vi "Batchify All Data.vi"(10 "Data":dbl[][](array[numeric])) -> (2 "Data Out":dbl[][](array[numeric]))   [LabVIEW 2013]
uses:
  Global Data/Names/Source Group Type.ctl
  Offsets Widget/Cartesian Or Actuator.ctl
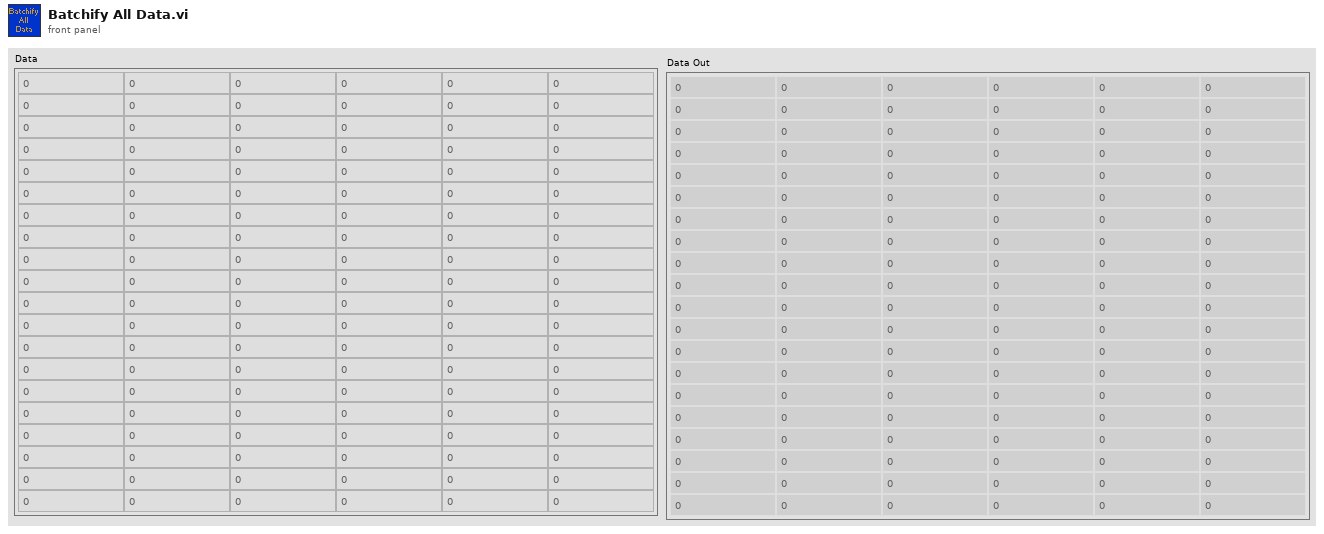
[diagram p1: front panel]
types:
  T1 = typedef "Source Group Type.ctl" = enum16{"LBCB1", "LBCB2", "Consolidated", "External"}
  T2 = typedef "Cartesian Or Actuator.ctl" = bool
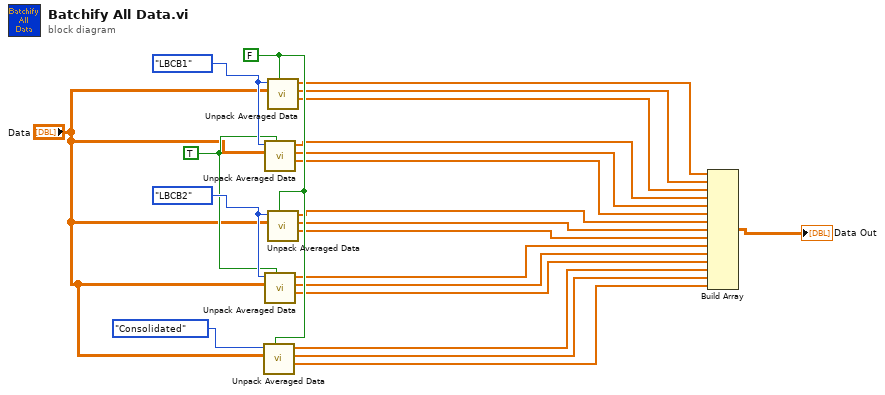
[diagram p0: block diagram]
diagram:
  w21 = Source_Group_Type."LBCB2" ("Source Group")
  w20 = T2 TRUE ("Coordinate Space")
  w18 = T2 FALSE ("Coordinate Space")
  w22 = Source_Group_Type."LBCB1" ("Source Group")
  n1 = call "Unpack Averaged Data.vi"("Coordinate Space"=w18, "Data"="Data", "Source Group"=Source_Group_Type."Consolidated") -> ("Forces"=w2:dbl[], "Disp"=w3:dbl[], "Cmds"=w4:dbl[])  [unwired: 6 in]
  n2 = call "Unpack Averaged Data.vi"("Coordinate Space"=w20, "Data"="Data", "Source Group"=w22) -> ("Forces"=w11:dbl[], "Disp"=w12:dbl[], "Cmds"=w13:dbl[])  [unwired: 6 in]
  n3 = call "Unpack Averaged Data.vi"("Coordinate Space"=w20, "Data"="Data", "Source Group"=w21) -> ("Forces"=w5:dbl[], "Disp"=w6:dbl[], "Cmds"=w7:dbl[])  [unwired: 6 in]
  n4 = call "Unpack Averaged Data.vi"("Coordinate Space"=w18, "Data"="Data", "Source Group"=w22) -> ("Forces"=w14:dbl[], "Disp"=w15:dbl[], "Cmds"=w16:dbl[])  [unwired: 6 in]
  n5 = call "Unpack Averaged Data.vi"("Coordinate Space"=w18, "Data"="Data", "Source Group"=w21) -> ("Forces"=w8:dbl[], "Disp"=w9:dbl[], "Cmds"=w10:dbl[])  [unwired: 6 in]
  n6 = Build Array(w16, w15, w14, w13, w12, w11, w10, w9, w8, w7, w6, w5, w4, w3, w2) -> (→"Data Out":dbl[][])
